vi "TouchPanel.DatetimeGui.vi"(0 "num date/time in (now)":dbl=-1.0 format="%.2f") -> (4 "num date/time out":dbl=3018608562.1229997 format="%.2f", 8 "ok":bool)   [LabVIEW 2016]
uses:
  Translator/Translator.Global.vi
panel:
  in  "SetTimeToNowButton":bool caption="OKButton"
  out "Sunday":bool
  out "Saturday":bool
  out "Friday":bool
  out "Thursday":bool
  out "Wednesday":bool
  out "Tuesday":bool
  out "Monday":bool
  in  "seconds":i32 min=0 max=59 format="%0#2_2d"
  in  "minutes":i32 min=0 max=59 format="%0#2_2d"
  in  "hour":i32 min=0 max=23 format="%0#2_2d"
  in  "CancelButton":bool
  in  "OKButton":bool
  in  "~b 1":bool=TRUE
  in  "~b 31":bool
  in  "~b 30":bool
  in  "~b 29":bool
  in  "~b 28":bool
  in  "~b 27":bool
  in  "~b 26":bool
  in  "~b 25":bool
  in  "~b 24":bool
  in  "~b 23":bool
  in  "~b 22":bool
  in  "~b 21":bool
  in  "~b 20":bool
  in  "~b 19":bool
  in  "~b 18":bool
  in  "~b 17":bool
  in  "~b 16":bool
  in  "~b 15":bool
  in  "~b 14":bool
  in  "~b 13":bool
  in  "~b 12":bool
  in  "~b 11":bool
  in  "~b 10":bool
  in  "~b 9":bool
  in  "~b 8":bool
  in  "~b 7":bool
  in  "~b 6":bool
  in  "~b 5":bool
  in  "~b 4":bool
  in  "~b 3":bool
  in  "~b 2":bool
  in  "Year":i32=2000 min=1904 max=2040 step=1
  out "?":string
  in  "Month":u16(ring) items=["January", "February", "March", "April", "May", "June", "July", "August", "September", "October", "November", "December"]
  # ":"
  # ":"
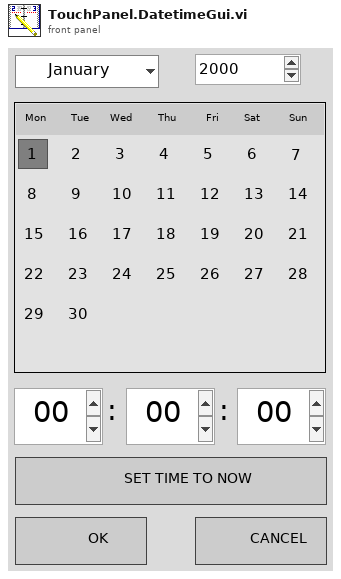
[diagram p1: front panel]
types:
  T1 = cluster{"second":i32, "minute":i32, "hour":i32, "day of month":i32, "month":i32, "year":i32, "day of week":i32, "day of year":i32, "is DST":i32}
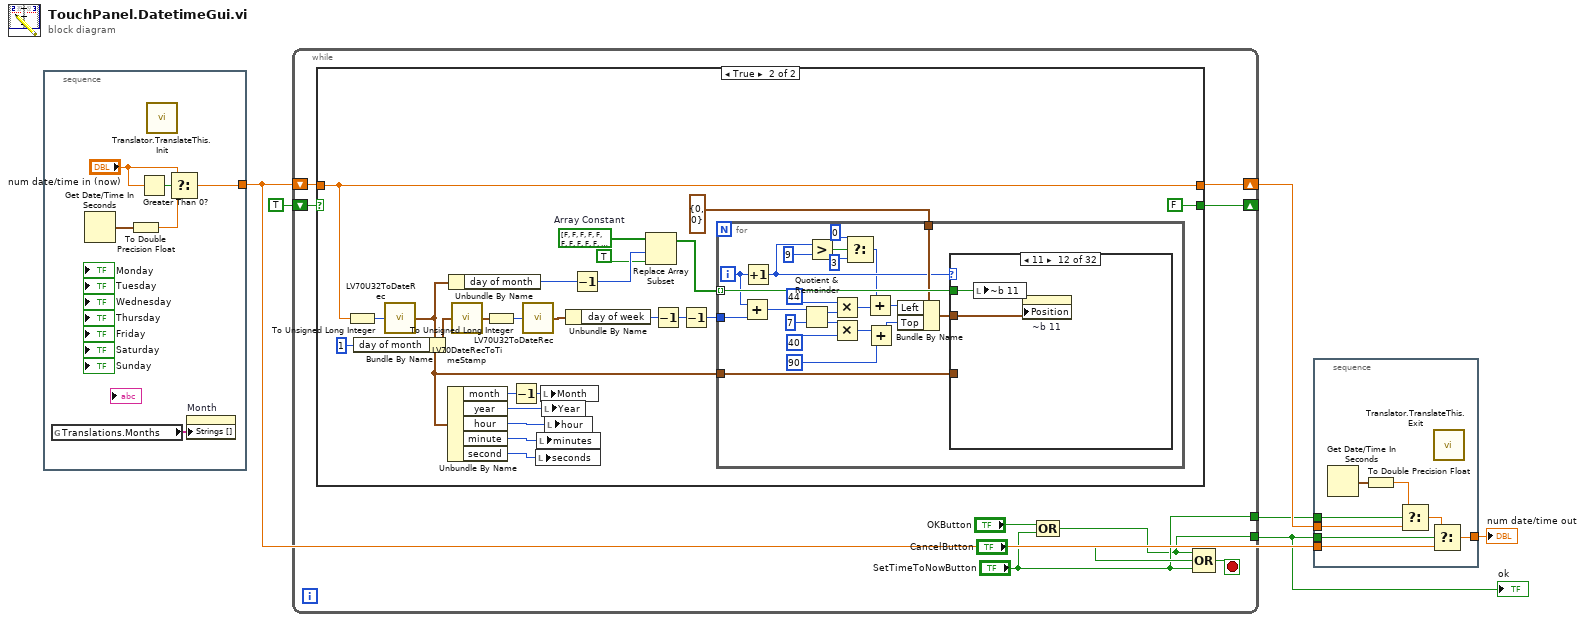
[diagram p0: block diagram]
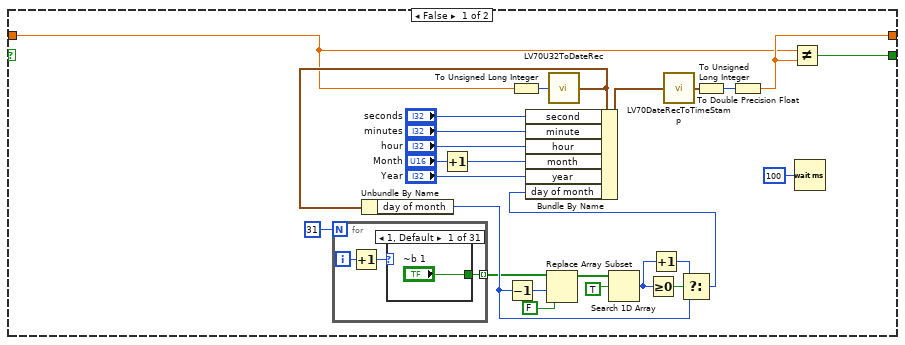
[diagram p2: hidden frame]
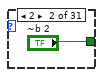
[diagram p3: hidden frame]
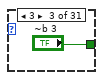
[diagram p4: hidden frame]
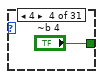
[diagram p5: hidden frame]
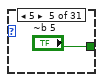
[diagram p6: hidden frame]
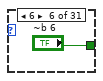
[diagram p7: hidden frame]
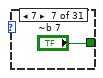
[diagram p8: hidden frame]
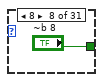
[diagram p9: hidden frame]
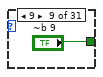
[diagram p10: hidden frame]
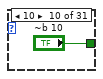
[diagram p11: hidden frame]
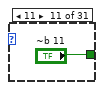
[diagram p12: hidden frame]
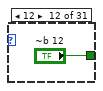
[diagram p13: hidden frame]
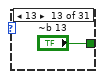
[diagram p14: hidden frame]
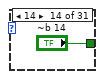
[diagram p15: hidden frame]
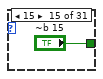
[diagram p16: hidden frame]
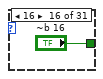
[diagram p17: hidden frame]
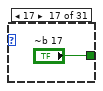
[diagram p18: hidden frame]
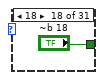
[diagram p19: hidden frame]
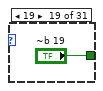
[diagram p20: hidden frame]
diagram:
  n1 = stacked-sequence {
    tunnel: [w8] -> w5
    frame #0 {
      n2 = global read "Translator.Global.vi" "Translations.Months"() -> (w11:string[])
      n3 = Get Date/Time In Seconds() -> (seconds since 1Jan1904=w7:timestamp)
      n4 = To Double Precision Float(number=w7) -> (double precision float=w12:dbl)
      n5 = Greater Than 0?(x="num date/time in (now)") -> (x > 0?=w10:bool)
      n6 = call "Translator.TranslateThis.Init.vi"() -> ()  [unwired: 11 in, 1 out]
      n7 = Select(t="num date/time in (now)", s=w10, f=w12) -> (s? t:f=w8:dbl)
      n8 = property on="Month" class="Ring (strict)"("Strings []"=w11) -> ()  [unwired: 2 in, 2 out]
    }
  }
  n9 = while {
    shift-left: TRUE -> [w16]
    shift-right: [w19] -> _
    tunnel: [w13] -> w1
    shift-left: w5 -> [w17]
    shift-right: [w21] -> w4
    tunnel: ["SetTimeToNowButton"] -> w3
    stop <- w20 stop-if-true
    n10 = case shown="True" w16 {
      tunnel: [w25 w105] -> w21
      tunnel: w17 -> [w24 w105]
      tunnel: [w23 FALSE] -> w19
      frame False {
        n11 = for {
          N: 31 -> [_]
          tunnel: [w48] -> w31 mode=indexing
          i -> [w50]
          n12 = Increment(x=w50) -> (x+1=w49:i32)
          n13 = case shown="1, Default" w49 {
            tunnel: ["~b 1" "~b 2" "~b 3" "~b 4" "~b 5" "~b 6" "~b 7" "~b 8" "~b 9" "~b 10" "~b 11" "~b 12" "~b 13" "~b 14" "~b 15" "~b 16" "~b 17" "~b 18" "~b 19" "~b 20" "~b 21" "~b 22" "~b 23" "~b 24" "~b 25" "~b 26" "~b 27" "~b 28" "~b 29" "~b 30" "~b 31"] -> w48
            frame 1, Default {
            }
            frame 2 {
            }
            frame 3 {
            }
            frame 4 {
            }
            frame 5 {
            }
            frame 6 {
            }
            frame 7 {
            }
            frame 8 {
            }
            frame 9 {
            }
            frame 10 {
            }
            frame 11 {
            }
            frame 12 {
            }
            frame 13 {
            }
            frame 14 {
            }
            frame 15 {
            }
            frame 16 {
            }
            frame 17 {
            }
            frame 18 {
            }
            frame 19 {
            }
            frame 20 {
            }
            frame 21 {
            }
            frame 22 {
            }
            frame 23 {
            }
            frame 24 {
            }
            frame 25 {
            }
            frame 26 {
            }
            frame 27 {
            }
            frame 28 {
            }
            frame 29 {
            }
            frame 30 {
            }
            frame 31 {
            }
          }
        }
        n14 = Increment(x="Month") -> (x+1=w29:u16)
        n15 = To Unsigned Long Integer(number=w24) -> (unsigned 32bit integer=w45:u32)
        n16 = call <vilib>:"LV70U32ToDateRec.vi"("Time"=w45) -> ("date time rec"=w34:T1)
        n17 = Unbundle By Name(w34) -> ("day of month"=w38:i32)
        n18 = Decrement(x=w38) -> (x-1=w40:i32)
        n19 = Replace Array Subset(array=w31, new element=FALSE ("Element Data"), index=w40) -> (w39:bool[])
        n20 = Search 1D Array(1D array=w39, element=TRUE ("Element Data")) -> (index of element=w37:i32)  [unwired: 1 out]
        n21 = Greater Or Equal To 0?(x=w37) -> (x >= 0?=w33:bool)
        n22 = Increment(x=w37) -> (x+1=w36:i32)
        n23 = Select(t=w36, s=w33, f=w38) -> (s? t:f=w35:i32)
        n24 = Bundle By Name(cluster=w34, "second"="seconds", "minute"="minutes", "hour"="hour", "month"=w29, "year"="Year", "day of month"=w35) -> (w46:T1)
        n25 = call <vilib>:"LV70DateRecToTimeStamp.vi"("date time rec"=w46) -> ("Time Stamp"=w30:timestamp)
        n26 = To Unsigned Long Integer(number=w30) -> (unsigned 32bit integer=w43:u32)
        n27 = To Double Precision Float(number=w43) -> (double precision float=w25:dbl)
        n28 = Not Equal?(x=w24, y=w25) -> (x != y?=w23:bool)
        n29 = Wait (ms)(milliseconds to wait=u32 100) -> ()  [unwired: 1 out]
      }
      frame True {
        w97 = bool[] [FALSE, FALSE, FALSE, FALSE, FALSE, FALSE, FALSE, FALSE, FALSE, FALSE, FALSE, FALSE, FALSE, FALSE, FALSE, FALSE, FALSE, FALSE, FALSE, FALSE, FALSE, FALSE, FALSE, FALSE, FALSE, FALSE, FALSE, FALSE, FALSE, FALSE, FALSE]  # Array Constant
        n30 = To Unsigned Long Integer(number=w105) -> (unsigned 32bit integer=w89:u32)
        n31 = call <vilib>:"LV70U32ToDateRec.vi"("Time"=w89) -> ("date time rec"=w87:T1)
        n32 = Bundle By Name(cluster=w87, "day of month"=1 ("Bundle Element")) -> (w91:T1)
        n33 = Unbundle By Name(w87) -> ("month"=w102:i32, "year"=w88:i32, "hour"=w84:i32, "minute"=w83:i32, "second"=w82:i32)
        n34 = Unbundle By Name(w87) -> ("day of month"=w100:i32)
        n35 = call <vilib>:"LV70DateRecToTimeStamp.vi"("date time rec"=w91) -> ("Time Stamp"=w92:timestamp)
        n36 = To Unsigned Long Integer(number=w92) -> (unsigned 32bit integer=w86:u32)
        n37 = Decrement(x=w102) -> (x-1=w103:i32)
        n38 = call <vilib>:"LV70U32ToDateRec.vi"("Time"=w86) -> ("date time rec"=w93:T1)
        n39 = local write "seconds"(w82) -> ()
        n40 = local write "minutes"(w83) -> ()
        n41 = local write "Month"(w103) -> ()
        n42 = local write "Year"(w88) -> ()
        n43 = local write "hour"(w84) -> ()
        n44 = Unbundle By Name(w93) -> ("day of week"=w94:i32)
        n45 = Decrement(x=w100) -> (x-1=w101:i32)
        n46 = Replace Array Subset(array=w97, new element=TRUE ("Element Data"), index=w101) -> (w98:bool[])
        n47 = Decrement(x=w94) -> (x-1=w85:i32)
        n48 = Decrement(x=w85) -> (x-1=w96:i32)
        n49 = for {
          tunnel: w98 -> [w128] mode=indexing
          tunnel: w96 -> [w113]
          tunnel: cluster{"Left":u32, "Top":u32} {"Left"=0, "Top"=0} ("Write Attribute") -> [w124]
          tunnel: w87 -> [w106]
          i -> [w127]
          n50 = Add(x=w127, y=w113) -> (x+y=w126:i32)
          n51 = Increment(x=w127) -> (x+1=w111:i32)
          n52 = Quotient & Remainder(x=w126, y=7) -> (x-y*floor(x/y)=w123:i32, floor(x/y)=w122:i32)
          n53 = Greater?(x=w111, y=9) -> (0:w110:bool)
          n54 = Multiply(x=44 ("y"), y=w123) -> (x*y=w118:i32)
          n55 = Multiply(x=w122, y=40) -> (x*y=w116:i32)
          n56 = Select(t=0 ("y"), s=w110, f=3 ("y")) -> (s? t:f=w109:i32)
          n57 = Add(x=w109, y=w118) -> (x+y=w117:i32)
          n58 = Add(x=w116, y=90) -> (x+y=w115:i32)
          n59 = Bundle By Name(cluster=w124, "Left"=w117, "Top"=w115) -> (w119:cluster{"Left":u32, "Top":u32})
          n60 = case shown="11" w111 {
            selector: w111 -> [_ _ _ _ _ _ _ _ _ _ _ _ _ _ _ _ _ _ _ _ _ _ _ _ _ _ _ _ _ w187 w197 w208]
            tunnel: w128 -> [w130 _ w132 w134 w136 w138 w140 w142 w144 w146 w148 w150 w152 w154 w156 w158 w160 w162 w164 w166 w168 w170 w172 w174 w176 w178 w180 w182 w184 w194 w204 w214]
            tunnel: w119 -> [w129 _ w131 w133 w135 w137 w139 w141 w143 w145 w147 w149 w151 w153 w155 w157 w159 w161 w163 w165 w167 w169 w171 w173 w175 w177 w179 w181 w183 w193 w203 w213]
            tunnel: w106 -> [_ _ _ _ _ _ _ _ _ _ _ _ _ _ _ _ _ _ _ _ _ _ _ _ _ _ _ _ _ w188 w198 w206]
            frame 1 {
              n61 = local write "~b 1"(w130) -> ()
              n62 = property on="~b 1" class="Bool (strict)"("Position"=w129) -> ()  [unwired: 2 in, 2 out]
            }
            frame Default {
            }
            frame 2 {
              n63 = local write "~b 2"(w132) -> ()
              n64 = property on="~b 2" class="Bool (strict)"("Position"=w131) -> ()  [unwired: 2 in, 2 out]
            }
            frame 3 {
              n65 = local write "~b 3"(w134) -> ()
              n66 = property on="~b 3" class="Bool (strict)"("Position"=w133) -> ()  [unwired: 2 in, 2 out]
            }
            frame 4 {
              n67 = local write "~b 4"(w136) -> ()
              n68 = property on="~b 4" class="Bool (strict)"("Position"=w135) -> ()  [unwired: 2 in, 2 out]
            }
            frame 5 {
              n69 = local write "~b 5"(w138) -> ()
              n70 = property on="~b 5" class="Bool (strict)"("Position"=w137) -> ()  [unwired: 2 in, 2 out]
            }
            frame 6 {
              n71 = local write "~b 6"(w140) -> ()
              n72 = property on="~b 6" class="Bool (strict)"("Position"=w139) -> ()  [unwired: 2 in, 2 out]
            }
            frame 7 {
              n73 = local write "~b 7"(w142) -> ()
              n74 = property on="~b 7" class="Bool (strict)"("Position"=w141) -> ()  [unwired: 2 in, 2 out]
            }
            frame 8 {
              n75 = local write "~b 8"(w144) -> ()
              n76 = property on="~b 8" class="Bool (strict)"("Position"=w143) -> ()  [unwired: 2 in, 2 out]
            }
            frame 9 {
              n77 = local write "~b 9"(w146) -> ()
              n78 = property on="~b 9" class="Bool (strict)"("Position"=w145) -> ()  [unwired: 2 in, 2 out]
            }
            frame 10 {
              n79 = local write "~b 10"(w148) -> ()
              n80 = property on="~b 10" class="Bool (strict)"("Position"=w147) -> ()  [unwired: 2 in, 2 out]
            }
            frame 11 {
              n81 = local write "~b 11"(w150) -> ()
              n82 = property on="~b 11" class="Bool (strict)"("Position"=w149) -> ()  [unwired: 2 in, 2 out]
            }
            frame 12 {
              n83 = local write "~b 12"(w152) -> ()
              n84 = property on="~b 12" class="Bool (strict)"("Position"=w151) -> ()  [unwired: 2 in, 2 out]
            }
            frame 13 {
              n85 = local write "~b 13"(w154) -> ()
              n86 = property on="~b 13" class="Bool (strict)"("Position"=w153) -> ()  [unwired: 2 in, 2 out]
            }
            frame 14 {
              n87 = local write "~b 14"(w156) -> ()
              n88 = property on="~b 14" class="Bool (strict)"("Position"=w155) -> ()  [unwired: 2 in, 2 out]
            }
            frame 15 {
              n89 = local write "~b 15"(w158) -> ()
              n90 = property on="~b 15" class="Bool (strict)"("Position"=w157) -> ()  [unwired: 2 in, 2 out]
            }
            frame 16 {
              n91 = local write "~b 16"(w160) -> ()
              n92 = property on="~b 16" class="Bool (strict)"("Position"=w159) -> ()  [unwired: 2 in, 2 out]
            }
            frame 17 {
              n93 = local write "~b 17"(w162) -> ()
              n94 = property on="~b 17" class="Bool (strict)"("Position"=w161) -> ()  [unwired: 2 in, 2 out]
            }
            frame 18 {
              n95 = local write "~b 18"(w164) -> ()
              n96 = property on="~b 18" class="Bool (strict)"("Position"=w163) -> ()  [unwired: 2 in, 2 out]
            }
            frame 19 {
              n97 = local write "~b 19"(w166) -> ()
              n98 = property on="~b 19" class="Bool (strict)"("Position"=w165) -> ()  [unwired: 2 in, 2 out]
            }
            frame 20 {
              n99 = local write "~b 20"(w168) -> ()
              n100 = property on="~b 20" class="Bool (strict)"("Position"=w167) -> ()  [unwired: 2 in, 2 out]
            }
            frame 21 {
              n101 = local write "~b 21"(w170) -> ()
              n102 = property on="~b 21" class="Bool (strict)"("Position"=w169) -> ()  [unwired: 2 in, 2 out]
            }
            frame 22 {
              n103 = local write "~b 22"(w172) -> ()
              n104 = property on="~b 22" class="Bool (strict)"("Position"=w171) -> ()  [unwired: 2 in, 2 out]
            }
            frame 23 {
              n105 = local write "~b 23"(w174) -> ()
              n106 = property on="~b 23" class="Bool (strict)"("Position"=w173) -> ()  [unwired: 2 in, 2 out]
            }
            frame 24 {
              n107 = local write "~b 24"(w176) -> ()
              n108 = property on="~b 24" class="Bool (strict)"("Position"=w175) -> ()  [unwired: 2 in, 2 out]
            }
            frame 25 {
              n109 = local write "~b 25"(w178) -> ()
              n110 = property on="~b 25" class="Bool (strict)"("Position"=w177) -> ()  [unwired: 2 in, 2 out]
            }
            frame 26 {
              n111 = local write "~b 26"(w180) -> ()
              n112 = property on="~b 26" class="Bool (strict)"("Position"=w179) -> ()  [unwired: 2 in, 2 out]
            }
            frame 27 {
              n113 = local write "~b 27"(w182) -> ()
              n114 = property on="~b 27" class="Bool (strict)"("Position"=w181) -> ()  [unwired: 2 in, 2 out]
            }
            frame 28 {
              n115 = local write "~b 28"(w184) -> ()
              n116 = property on="~b 28" class="Bool (strict)"("Position"=w183) -> ()  [unwired: 2 in, 2 out]
            }
            frame 29 {
              n117 = local write "~b 29"(w194) -> ()
              n118 = Bundle By Name(cluster=w188, "day of month"=w187) -> (w189:T1)
              n119 = call <vilib>:"LV70DateRecToTimeStamp.vi"("date time rec"=w189) -> ("Time Stamp"=w185:timestamp)
              n120 = To Unsigned Long Integer(number=w185) -> (unsigned 32bit integer=w190:u32)
              n121 = call <vilib>:"LV70U32ToDateRec.vi"("Time"=w190) -> ("date time rec"=w191:T1)
              n122 = Unbundle By Name(w191) -> ("day of month"=w192:i32)
              n123 = Equal?(x=w187, y=w192) -> (x = y?=w186:bool)
              n124 = property on="~b 29" class="Bool (strict)"("Position"=w193, "Visible"=w186) -> ()  [unwired: 2 in, 2 out]
            }
            frame 30 {
              n125 = local write "~b 30"(w204) -> ()
              n126 = Bundle By Name(cluster=w198, "day of month"=w197) -> (w199:T1)
              n127 = call <vilib>:"LV70DateRecToTimeStamp.vi"("date time rec"=w199) -> ("Time Stamp"=w195:timestamp)
              n128 = To Unsigned Long Integer(number=w195) -> (unsigned 32bit integer=w200:u32)
              n129 = call <vilib>:"LV70U32ToDateRec.vi"("Time"=w200) -> ("date time rec"=w201:T1)
              n130 = Unbundle By Name(w201) -> ("day of month"=w202:i32)
              n131 = Equal?(x=w197, y=w202) -> (x = y?=w196:bool)
              n132 = property on="~b 30" class="Bool (strict)"("Position"=w203, "Visible"=w196) -> ()  [unwired: 2 in, 2 out]
            }
            frame 31 {
              n133 = Bundle By Name(cluster=w206, "day of month"=w208) -> (w209:T1)
              n134 = local write "~b 31"(w214) -> ()
              n135 = call <vilib>:"LV70DateRecToTimeStamp.vi"("date time rec"=w209) -> ("Time Stamp"=w205:timestamp)
              n136 = To Unsigned Long Integer(number=w205) -> (unsigned 32bit integer=w210:u32)
              n137 = call <vilib>:"LV70U32ToDateRec.vi"("Time"=w210) -> ("date time rec"=w211:T1)
              n138 = Unbundle By Name(w211) -> ("day of month"=w212:i32)
              n139 = Equal?(x=w208, y=w212) -> (x = y?=w207:bool)
              n140 = property on="~b 31" class="Bool (strict)"("Position"=w213, "Visible"=w207) -> ()  [unwired: 2 in, 2 out]
            }
          }
        }
      }
    }
    n141 = Compound Arithmetic op=OR("OKButton", "SetTimeToNowButton") -> (w13:bool)
    n142 = Compound Arithmetic op=OR(w13, "CancelButton", "SetTimeToNowButton") -> (w20:bool)
  }
  "ok" <- w1
  n143 = stacked-sequence {
    tunnel: [w222] -> w2
    tunnel: w5 -> [w221]
    tunnel: w3 -> [w220]
    tunnel: w4 -> [w219]
    tunnel: w1 -> [w217]
    frame #0 {
      n144 = Get Date/Time In Seconds() -> (seconds since 1Jan1904=w218:timestamp)
      n145 = To Double Precision Float(number=w218) -> (double precision float=w215:dbl)
      n146 = Select(t=w215, s=w220, f=w219) -> (s? t:f=w216:dbl)
      n147 = Select(t=w216, s=w217, f=w221) -> (s? t:f=w222:dbl)
      n148 = call "Translator.TranslateThis.Exit.vi"() -> ()  [unwired: 11 in, 1 out]
    }
  }
  "num date/time out" <- w2
